vi "Load Animated GIF Image (Path).vi"(8 "error in (no error)":errorcluster, 11 "Path In":path) -> (0 "error out":errorcluster, 1 "Delays":i32[](array[numeric]), 2 "Frames":T1[](array[typedef]), 3 "Path Out":path)   [LabVIEW 2020, in "G-Image.lvlib"]
doc: "Load an animated GIF image file from disk and return it as an array of LabVIEW pictures.\n\nThe Delays array are the time in milliseconds to display each frame, and can vary between frames.\n\nNote this function can load non-animated GIF types, which are returned as a single frame."
uses:
  G-Image.lvlib
  <vilib>/picture/picture.llb/imagedata.ctl
  Private/Result To Error.vi
  <vilib>/Utility/error.llb/Error Cluster From Error Code.vi
  Private/Copy Image To Picture.vi
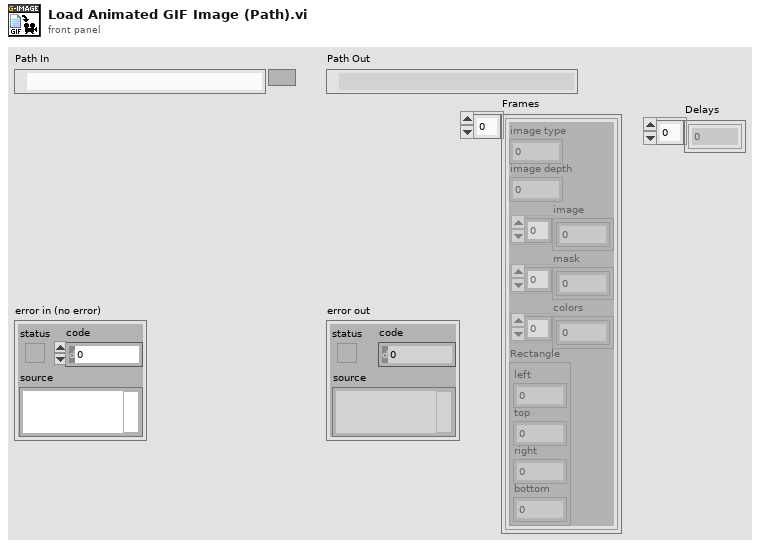
[diagram p1: front panel]
types:
  T1 = typedef "imagedata.ctl" = cluster{"image type":i32, "image depth":i32, "image":u8[], "mask":u8[], "colors":u32[], "Rectangle":cluster{"left":i16, "top":i16, "right":i16, "bottom":i16}}
  T2 = typedef "G-Image.lvlib/Extended Image.ctl" = cluster{"Image":T1, "Layers":i32, "Delays":i32[]}
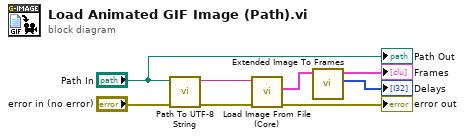
[diagram p0: block diagram]
diagram:
  n1 = call "Path To UTF-8 String.vi"("error in"="error in (no error)", "Path"="Path In") -> ("error out"=w4:errorcluster, "UTF-8 String"=w7:string)  [unwired: 8 in]
  n2 = call "Load Image From File (Core).vi"("error in (no error)"=w4, "Path In"=w7) -> ("error out"=→"error out":errorcluster, "Extended Image"=w3:T2)  [unwired: 7 in, 1 out]
  n3 = call "Extended Image To Frames.vi"("Extended Image"=w3) -> ("Delays"=→"Delays":i32[], "Frames"=→"Frames":T1[])  [unwired: 9 in]
  "Path Out" <- "Path In"
